vi "CameraAttributeSearch.vi"() -> ()   [LabVIEW 2024]
uses:
  <vilib>/userDefined/High Color/IMAQdx.ctl
  <vilib>/vision/driver/IMAQdx.llb/IMAQdx Attribute Type.ctl
  <vilib>/regexp/Match Regular Expression.xnode
  <vilib>/vision/driver/NI_Vision_Acquisition_Software.lvlib
panel:
  out "Ready":bool=TRUE
  out "Array":T2(array[cluster])
  in  "Attribute search":string
  in  "stop":bool
  in  "Session In":T3
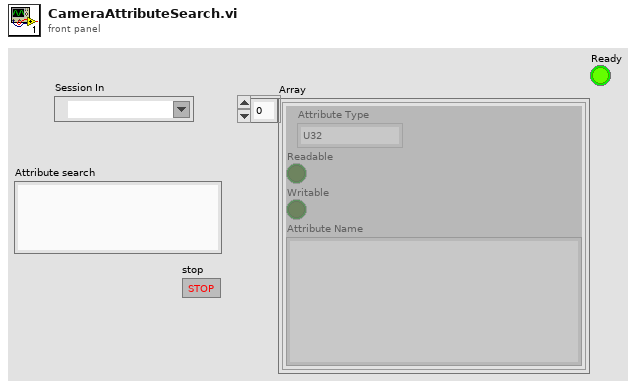
[diagram p1: front panel]
types:
  T1 = typedef "NI_Vision_Acquisition_Software.lvlib/IMAQdx Attribute Type.ctl" = enum32{"U32", "I64", "DBL", "String", "Enum", "Bool", "Command"}
  T2 = cluster{"Attribute Type":T1, "Readable":bool, "Writable":bool, "Attribute Name":string}[]
  T3 = typedef "IMAQdx.ctl" = refnum<k21>
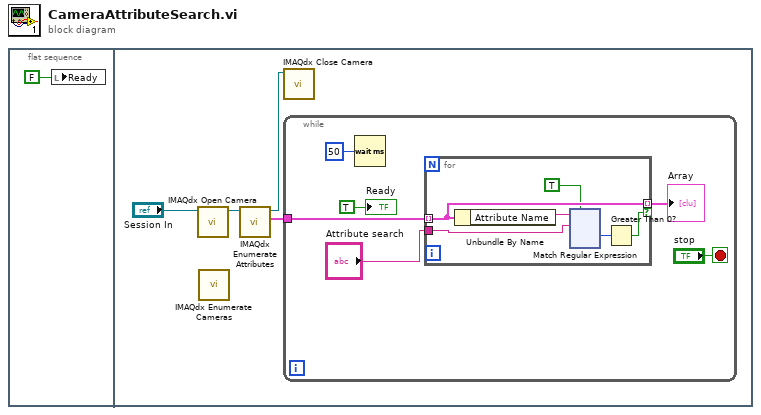
[diagram p0: block diagram]
diagram:
  n1 = flat-sequence {
    frame #0 {
      n2 = local write "Ready"(FALSE) -> ()
    }
    frame #1 {
      n3 = call <vilib>:"IMAQdx Open Camera.vi"("Session In"="Session In") -> ("Session Out"=w5:T3)  [unwired: 9 in, 1 out]
      n4 = call <vilib>:"IMAQdx Enumerate Cameras.vi"() -> ()  [unwired: 10 in, 2 out]
      n5 = call <vilib>:"IMAQdx Enumerate Attributes.vi"("Session In"=w5) -> ("Attribute Information Array"=w3:T2, "Session Out"=w4:T3)  [unwired: 8 in, 1 out]
      n6 = call <vilib>:"IMAQdx Close Camera.vi"("Session In"=w4) -> ()  [unwired: 10 in, 1 out]
      n7 = while {
        tunnel: w3 -> [w9]
        stop <- "stop" stop-if-true
        n8 = Wait (ms)(milliseconds to wait=u32 50) -> ()  [unwired: 1 out]
        n9 = for {
          tunnel: w9 -> [w16] mode=indexing
          tunnel: "Attribute search" -> [w15]
          tunnel: [w16] -> w7 mode=indexing if=w17
          n10 = Unbundle By Name(w16) -> ("Attribute Name"=w14:string)
          n11 = xnode "Match Regular Expression"("input string"=w14, "regular expression"=w15, "ignore case? (F)"=TRUE) -> ("offset past match"=w13:i32)  [unwired: 3 in, 4 out]
          n12 = Greater Than 0?(x=w13) -> (x > 0?=w17:bool)
        }
        "Array" <- w7
        "Ready" <- TRUE
      }
    }
  }
